vi "Invalid Configuration--error.vi"() -> (0 "error out":errorcluster)   [LabVIEW 2020, in "CICD.lvlib"]
doc: "Error configuration not valid."
uses:
  CICD.lvlib
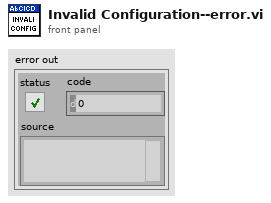
[diagram p1: front panel]
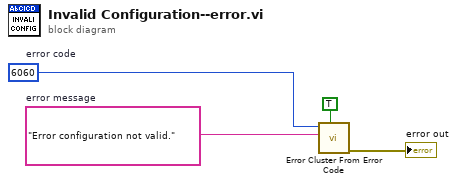
[diagram p0: block diagram]
diagram:
  w2 = "Error configuration not valid."  # error message
  w3 = 6060  # error code
  n1 = call <vilib>:"Error Cluster From Error Code.vi"("show call chain? (False)"=TRUE, "error message (\"\")"=w2, "error code (0)"=w3) -> ("error out"=→"error out":errorcluster)  [unwired: 6 in]
